vi "ParseResult.vi"(7 "VI Analyzer report path":path, 8 "error in (no error)":errorcluster, 11 "Summary Statistics":T1) -> (0 "error out":errorcluster, 1 "Output":string, 2 "Passed?":bool)   [LabVIEW 2014, in "RunVIAnalyzer.lvclass"]
uses:
  RunVIAnalyzer.lvclass
panel:
  in  "VI Analyzer Summary ouput":string="VI Analyzer completed.\\n%d tests passed.\\n%d tests failed.\\n%d tests skipped.\\n%d VIs were unloadable.\\n%d tests were unloadable.\\n%d tests were unrunable.\\n%d tests produced error.\\n\\nPlease find the full report at \"%s\"."
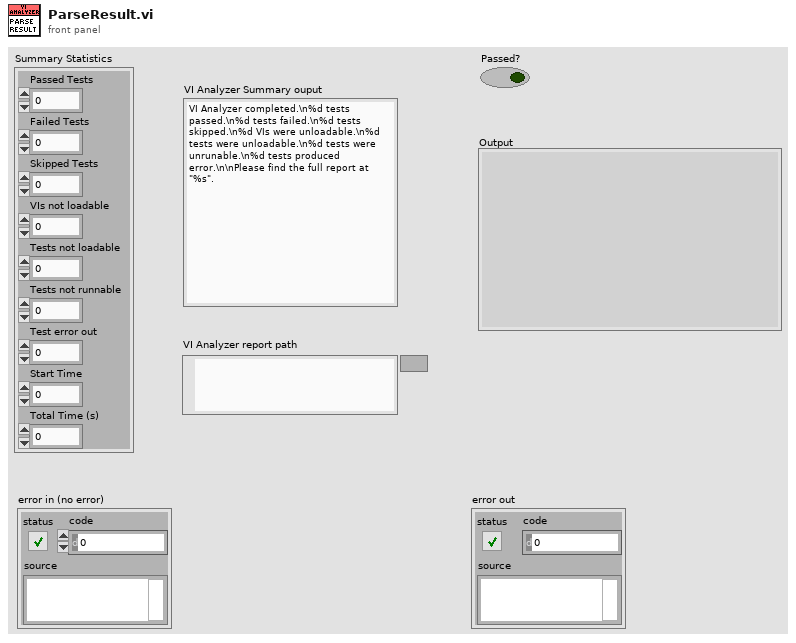
[diagram p1: front panel]
types:
  T1 = cluster{"Passed Tests":i32, "Failed Tests":i32, "Skipped Tests":i32, "VIs not loadable":i32, "Tests not loadable":i32, "Tests not runnable":i32, "Test error out":i32, "Start Time":u32, "Total Time (s)":dbl}
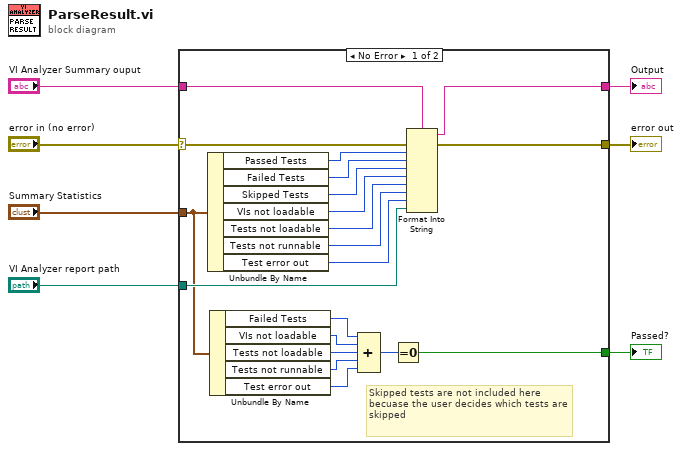
[diagram p0: block diagram]
diagram:
  n1 = case shown="No Error" "error in (no error)" {
    selector: "error in (no error)" -> [w26 w28]
    tunnel: "Summary Statistics" -> [w15 _]
    tunnel: [w25 w28] -> w6
    tunnel: [w16 _] -> w7
    tunnel: "VI Analyzer Summary ouput" -> [w27 _]
    tunnel: "VI Analyzer report path" -> [w17 _]
    tunnel: [w9 _] -> w1
    frame No Error {
      # "Skipped tests are not included here becuase the user decides which tests are skipped"
      n2 = Unbundle By Name(w15) -> ("Passed Tests"=w24:i32, "Failed Tests"=w23:i32, "Skipped Tests"=w22:i32, "VIs not loadable"=w21:i32, "Tests not loadable"=w20:i32, "Tests not runnable"=w19:i32, "Test error out"=w18:i32)
      n3 = Unbundle By Name(w15) -> ("Failed Tests"=w14:i32, "VIs not loadable"=w8:i32, "Tests not loadable"=w13:i32, "Tests not runnable"=w12:i32, "Test error out"=w11:i32)
      n4 = Compound Arithmetic op=ADD(w14, w8, w13, w12, w11) -> (w10:i32)
      n5 = Equal To 0?(x=w10) -> (x = 0?=w9:bool)
      n6 = Format Into String(format string=w27, error in=w26, w24, w23, w22, w21, w20, w19, w18, w17) -> (resulting string=w16:string, error out=w25:errorcluster)  [unwired: 1 in]
    }
    frame Error {
    }
  }
  "Output" <- w7
  "Passed?" <- w1
  "error out" <- w6
